vi "Arreglo_de_media_movil.vi"(6 "N":dbl, 9 "Numeric 3":i32, 10 "Numeric in":dbl, 11 "Array in":dbl[](array[numeric])) -> (2 "Numeric out":dbl, 3 "Array out":dbl[](array[numeric]))   [LabVIEW 2016]
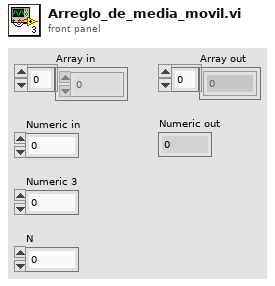
[diagram p1: front panel]
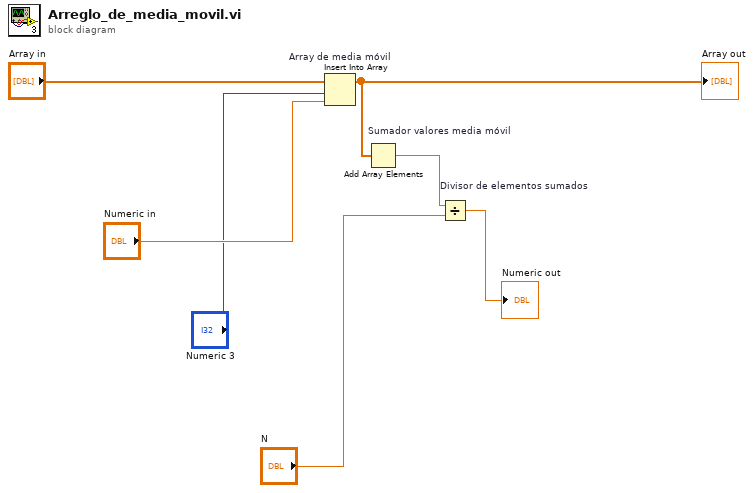
[diagram p0: block diagram]
diagram:
  n1 = Insert Into Array "Array de media móvil"(array="Array in", index="Numeric 3", new element="Numeric in") -> (w3:dbl[])
  "Array out" <- w3
  n2 = Add Array Elements "Sumador valores media móvil"(numeric array=w3) -> (sum=w6:dbl)
  n3 = Divide "Divisor de elementos sumados"(x=w6, y="N") -> (x/y=→"Numeric out":dbl)
